vi "Test UDP.vi"() -> ()   [LabVIEW 2014]
uses:
  myRIO/Controls/Switch Program.ctl
  myRIO/Controls/Action Enum.ctl
  myRIO/Controls/Switch Day.ctl
panel:
  in  "Switch Program":T1
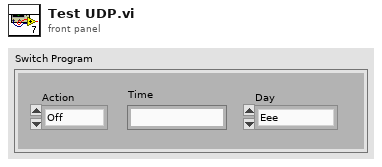
[diagram p1: front panel]
types:
  T1 = typedef "Switch Program.ctl" = cluster{"Action":T2, "Time":string, "Day":T3}
  T2 = typedef "Action Enum.ctl" = enum16{"Off", "On"}
  T3 = typedef "Switch Day.ctl" = enum16{"Eee", "Sun", "Mon", "Tue", "Wed", "Thu", "Fri", "Sat"}
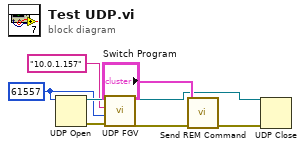
[diagram p0: block diagram]
diagram:
  w6 = u16 61557 ("port")
  n1 = UDP Open(11:w6) -> (port=w7:refnum<k16>, 0:w8:errorcluster)  [unwired: 4 in, 1 out]
  n2 = call "UDP FGV.vi"("error in (no error)"=w8, "Port"=w6, "IP Address"="10.0.1.157", "connection ID"=w7) -> ("error out"=w4:errorcluster, "connection ID out"=w1:refnum<k16>)  [unwired: 4 in, 2 out]
  n3 = call "Send REM Command.vi"("error in (no error)"=w4, "Switch Program"="Switch Program") -> ("error out"=w2:errorcluster)  [unwired: 9 in]
  n4 = UDP Close(connection ID=w1, 8:w2) -> ()  [unwired: 2 out]
